vi "Rysowanie skali mapy.vi"(7 "Rozmiar obszaru widocznej mapy":T1, 9 "Parametry":T2, 10 "Długość piksela w metrach":dbl=0.19634281539316645, 11 "Obraz wejściowy":picture) -> (3 "Obraz wyjściowy":picture)   [LabVIEW 2012, in "Biblioteka moduł map v3.lvlib" / "Obsługa grafiki mapy.lvlib"]
doc: "Zadaniem pliku jest dorysowanie do aktualnego obrazu mapy skali o zadanych parametrach z uwzględnieniem przesunięcia mapy."
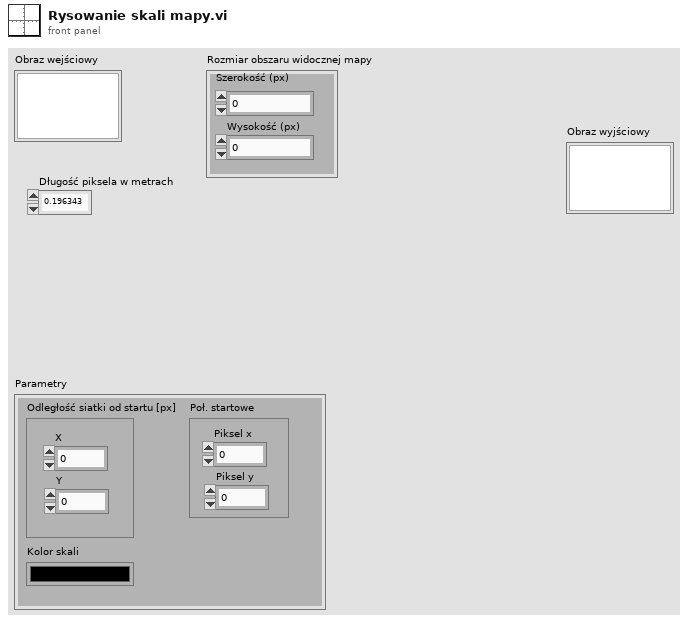
[diagram p1: front panel]
types:
  T1 = cluster{"Szerokość (px)":i16, "Wysokość (px)":i16}
  T2 = cluster{"Kolor skali":u32, "Odległość siatki od startu [px]":cluster{"X ":i32, "Y ":i32}, "Poł. startowe":cluster{"Piksel x":i32, "Piksel y":i32}}
  T3 = cluster{"coordinate 1":i16, "value 1":dbl, "coordinate 2":i16, "value 2":dbl, "log?(F)":bool, "fmt and prec":cluster{"format":enum8{"Decimal", "Scientific", "Engineering", "Binary", "Octal", "Hex"}, "precision":u8}}
  T4 = cluster{"horizontal":bool, "left/top":bool, "draw bar":bool, "line color":u32, "text color(black)":u32}
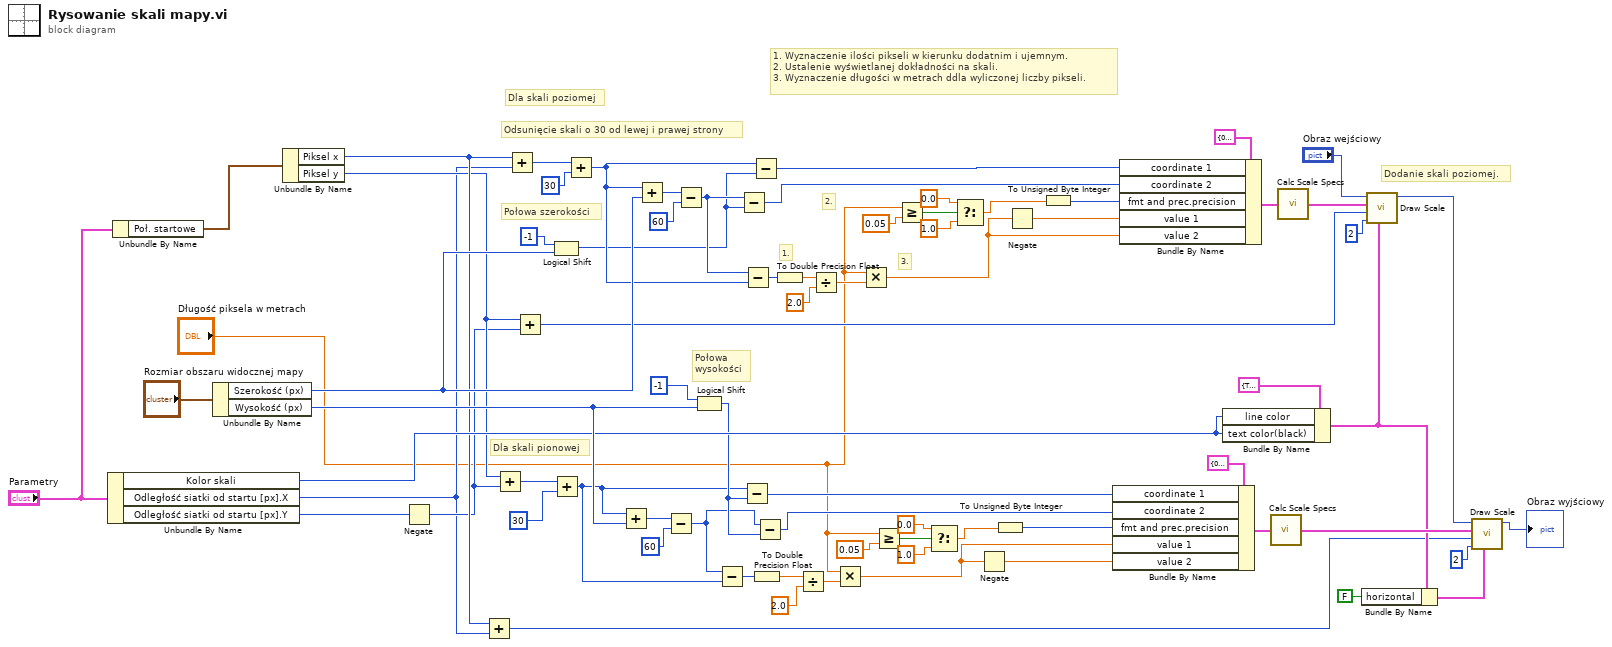
[diagram p0: block diagram]
diagram:
  # "Połowa\nwysokości"
  # "Połowa szerokości"
  # "Dla skali pionowej"
  # "Dla skali poziomej"
  # "2."
  # "3."
  # "1. Wyznaczenie ilości pikseli w kierunku dodatnim i ujemnym.\n2. Ustalenie wyświetlanej dokładności na skali.\n3. Wyznaczenie długości w metrach ddla wyliczonej liczby pikseli."
  # "1."
  # "Odsunięcie skali o 30 od lewej i prawej strony"
  # "Dodanie skali poziomej."
  n1 = Unbundle By Name("Parametry") -> ("Kolor skali"=w24:u32, "Odległość siatki od startu [px].X"=w4:i32, "Odległość siatki od startu [px].Y"=w3:i32)
  n2 = Unbundle By Name("Parametry") -> ("Poł. startowe"=w2:cluster{"Piksel x":i32, "Piksel y":i32})
  n3 = Unbundle By Name("Rozmiar obszaru widocznej mapy") -> ("Szerokość (px)"=w29:i16, "Wysokość (px)"=w26:i16)
  n4 = Unbundle By Name(w2) -> ("Piksel x"=w10:i32, "Piksel y"=w8:i32)
  n5 = Negate(x=w3) -> (-x=w6:i32)
  n6 = Add(x=w10, y=w4) -> (x+y=w9:i32)
  n7 = Add(x=w8, y=w6) -> (x+y=w47:i32)
  n8 = Add(x=w10, y=w4) -> (x+y=w38:i32)
  n9 = Add(x=w8, y=w6) -> (x+y=w7:i32)
  n10 = Logical Shift(y=i16 -1, x=w29) -> (x << y=w16:i16)
  n11 = Add(x=w47, y=i16 30) -> (x+y=w13:i32)
  n12 = Add(x=w38, y=i16 30) -> (x+y=w17:i32)
  n13 = Add(x=w13, y=w26) -> (x+y=w49:i32)
  n14 = Add(x=w17, y=w29) -> (x+y=w66:i32)
  n15 = Subtract(x=w49, y=i16 60) -> (x-y=w14:i32)
  n16 = Subtract(x=w66, y=i16 60) -> (x-y=w20:i32)
  n17 = Logical Shift(y=i16 -1, x=w26) -> (x << y=w15:i16)
  n18 = Subtract(x=w14, y=w13) -> (x-y=w33:i32)
  n19 = Subtract(x=w20, y=w16) -> (x-y=w19:i32)
  n20 = Subtract(x=w13, y=w15) -> (x-y=w11:i32)
  n21 = Subtract(x=w20, y=w17) -> (x-y=w37:i32)
  n22 = Subtract(x=w17, y=w16) -> (x-y=w18:i32)
  n23 = To Double Precision Float(number=w33) -> (double precision float=w32:dbl)
  n24 = Subtract(x=w14, y=w15) -> (x-y=w12:i32)
  n25 = To Double Precision Float(number=w37) -> (double precision float=w36:dbl)
  n26 = Divide(x=w32, y=2.0) -> (x/y=w52:dbl)
  n27 = Divide(x=w36, y=2.0) -> (x/y=w63:dbl)
  n28 = Multiply(x="Długość piksela w metrach", y=w52) -> (x*y=w39:dbl)
  n29 = Multiply(x="Długość piksela w metrach", y=w63) -> (x*y=w61:dbl)
  n30 = Greater Or Equal?(x="Długość piksela w metrach", y=0.05) -> (x >= y?=w54:bool)
  n31 = Greater Or Equal?(x="Długość piksela w metrach", y=0.05) -> (x >= y?=w59:bool)
  n32 = Select(t=0.0, s=w54, f=1.0) -> (s? t:f=w31:dbl)
  n33 = Select(t=0.0, s=w59, f=1.0) -> (s? t:f=w34:dbl)
  n34 = Negate(x=w39) -> (-x=w40:dbl)
  n35 = To Unsigned Byte Integer(number=w31) -> (unsigned 8bit integer=w30:u8)
  n36 = Negate(x=w61) -> (-x=w62:dbl)
  n37 = To Unsigned Byte Integer(number=w34) -> (unsigned 8bit integer=w35:u8)
  n38 = Bundle By Name(cluster=T3 {"coordinate 1"=0, "value 1"=-5.0, "coordinate 2"=5, "value 2"=5.0, "log?(F)"=FALSE, "fmt and prec"={"format"=enum."Decimal", "precision"=0}} ("scale definition"), "coordinate 1"=w11, "coordinate 2"=w12, "fmt and prec.precision"=w30, "value 1"=w39, "value 2"=w40) -> (w46:T3)
  n39 = Bundle By Name(cluster=T3 {"coordinate 1"=0, "value 1"=-5.0, "coordinate 2"=5, "value 2"=5.0, "log?(F)"=FALSE, "fmt and prec"={"format"=enum."Decimal", "precision"=0}} ("scale definition"), "coordinate 1"=w18, "coordinate 2"=w19, "fmt and prec.precision"=w35, "value 1"=w62, "value 2"=w61) -> (w68:T3)
  n40 = Bundle By Name(cluster=T4 {"horizontal"=TRUE, "left/top"=FALSE, "draw bar"=TRUE, "line color"=0, "text color(black)"=0} ("scale attributes"), "line color"=w24, "text color(black)"=w24) -> (w23:T4)
  n41 = call <vilib>:"Calc Scale Specs.vi"("scale definition"=w46) -> ("scale specs"=w43:cluster{"coordinate":i16, "label":string}[])  [unwired: 8 in]
  n42 = call <vilib>:"Calc Scale Specs.vi"("scale definition"=w68) -> ("scale specs"=w73:cluster{"coordinate":i16, "label":string}[])  [unwired: 8 in]
  n43 = Bundle By Name(cluster=w23, "horizontal"=FALSE) -> (w21:T4)
  n44 = call <vilib>:"Draw Scale.vi"("scale attributes"=w23, "tick length(3)"=i16 2, "constant coordinate"=w7, "scale specs"=w73, "picture"="Obraz wejściowy") -> ("new picture"=w42:picture)  [unwired: 6 in]
  n45 = call <vilib>:"Draw Scale.vi"("scale attributes"=w21, "tick length(3)"=i16 2, "constant coordinate"=w9, "scale specs"=w43, "picture"=w42) -> ("new picture"=→"Obraz wyjściowy":picture)  [unwired: 6 in]
